vi "Close.vi"(8 "error in (no error)":errorcluster, 11 "CSV Test Log in":refnum<class "CSV Test Log.lvclass">) -> (0 "error out":errorcluster, 3 "CSV Test Log out":refnum<class "CSV Test Log.lvclass">)   [LabVIEW 2015, in "CSV Test Log.lvclass"]
uses:
  CSV Test Log.lvclass
  CSV Test Log.lvclass/CSV Test Log.ctl
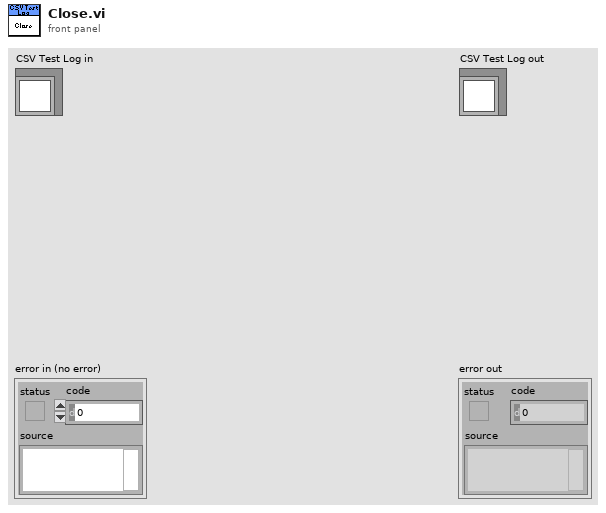
[diagram p1: front panel]
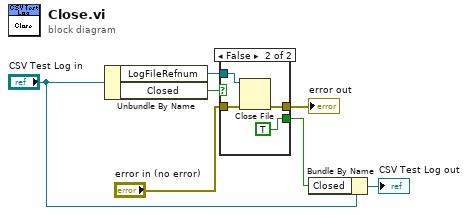
[diagram p0: block diagram]
diagram:
  n1 = Unbundle By Name("CSV Test Log in") -> ("LogFileRefnum"=w5:refnum<file>, "Closed"=w4:bool)
  n2 = case shown="False" w4 {
    selector: w4 -> [w8 _]
    tunnel: [w9 w13] -> w7
    tunnel: "error in (no error)" -> [w9 w12]
    tunnel: w5 -> [_ w11]
    tunnel: [w8 TRUE] -> w1
    frame True {
    }
    frame False {
      n3 = Close File(refnum=w11, error in=w12) -> (error out=w13:errorcluster)  [unwired: 1 out]
    }
  }
  "error out" <- w7
  n4 = Bundle By Name(cluster="CSV Test Log in", "Closed"=w1) -> (→"CSV Test Log out":refnum<class "CSV Test Log.lvclass">)
